vi "AttackerSmart.vi"(9 "balls":T1[](array[typedef])=[{"x"=-2165.869384765625, "y"=510.4085693359375, "timestamp"=timestamp(2082758857.4639893 s since 1904-01-01)}], 10 "Field Size in":T4={"line_width"=10, "field_length"=6000, "field_width"=4000, "boundary_width"=250, "referee_width"=425, "goal_width"=700, "goal_depth"=180, "goal_wall_width"=20, "center_circle_radius"=500, "defense_radius"=500, "defense_stretch"=350, "free_kick_from_defense_dist"=700, "penalty_spot_from_field_line_dist"=450, "penalty_line_from_spot_dist"=350}, 11 "Robot in":T2={"id"=5, "function"=enum."Attacker", "x"=-1842.5054931640625, "y"=520.60986328125, "orientation"=-2.7555055618286133, "v_tangent"=0.0, "v_normal"=0.0, "v_ang"=0.0, "kick_x"=0.0, "kick_z"=0.0, "dribble"=FALSE, "Timestamp"=timestamp(2082758857.4639893 s since 1904-01-01), "dest_x"=0.0, "dest_y"=0.0, "dest_orientation"=0.0}) -> (3 "Robot out":T2={"id"=5, "function"=enum."Attacker", "x"=-1842.5054931640625, "y"=520.60986328125, "orientation"=-2.7555055618286133, "v_tangent"=-0.08361641967936218, "v_normal"=-0.20513016702014014, "v_ang"=0.24456003022714357, "kick_x"=0.0, "kick_z"=0.0, "dribble"=FALSE, "Timestamp"=timestamp(2082758857.4639893 s since 1904-01-01), "dest_x"=0.0, "dest_y"=0.0, "dest_orientation"=0.0})   [LabVIEW 2016]
uses:
  Core/Field Size.ctl
  Core/AI Robot.ctl
  Functions Enum.ctl
  Core/AI Ball.ctl
  <vilib>/Analysis/coordinate.llb/Wrap Angle (scalar).vi
  <vilib>/Analysis/coordinate.llb/2D Cartesian Coordinate Rotation (Scalar).vi
  <vilib>/Analysis/NI_AALPro.lvlib
  <vilib>/Analysis/NI_AAL_Angle.lvlib
panel:
  in  "min ang to kick":dbl=0.09 format="%#_13g"
  in  "min dist to kick":dbl=195.0 format="%#_13g"
  in  "farback":dbl=330.0 format="%#_13g"
  in  "behind ball\ntarget aperture":dbl=0.3490658503988659 format="%#_13g"
  in  "conditional\nangle":dbl=0.45 format="%#_13g"
  in  "Kick Time":u32
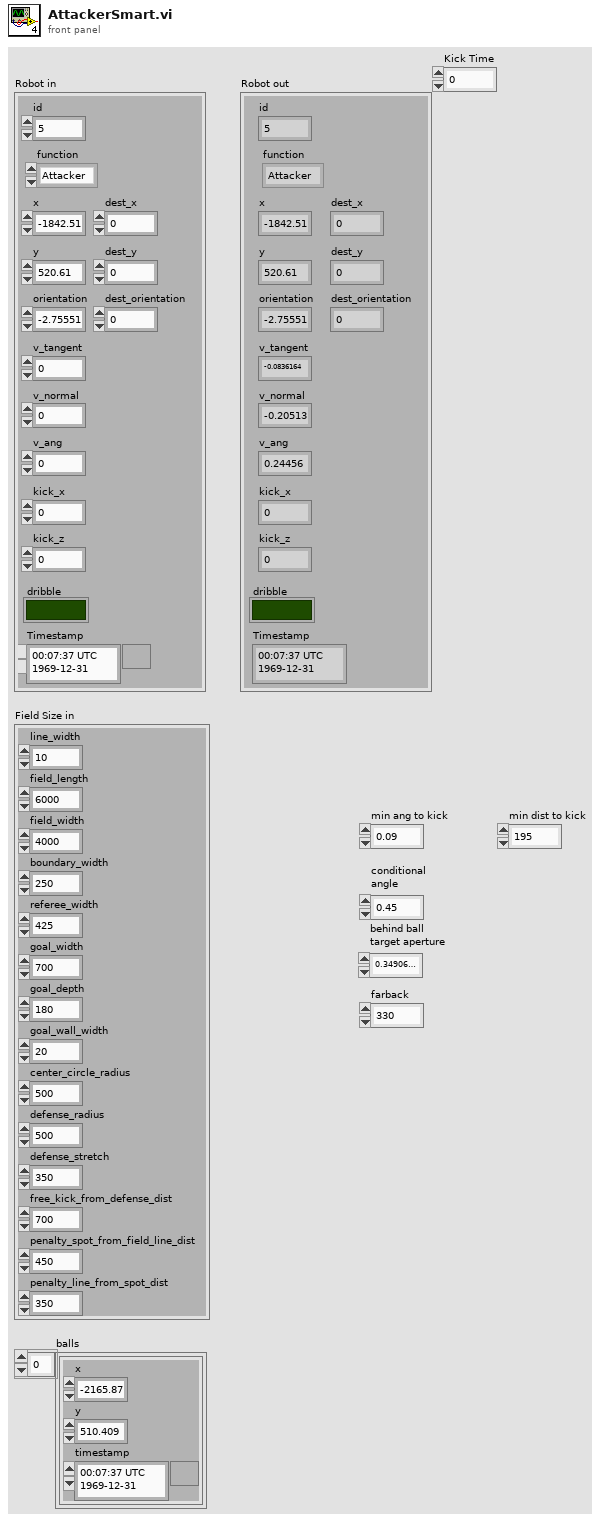
[diagram p1: front panel]
types:
  T1 = typedef "AI Ball.ctl" = cluster{"x":dbl, "y":dbl, "timestamp":timestamp}
  T2 = typedef "AI Robot.ctl" = cluster{"id":u32, "function":T3, "x":dbl, "y":dbl, "orientation":dbl, "v_tangent":dbl, "v_normal":dbl, "v_ang":dbl, "kick_x":dbl, "kick_z":dbl, "dribble":bool, "Timestamp":timestamp, "dest_x":dbl, "dest_y":dbl, "dest_orientation":dbl}
  T3 = typedef "Functions Enum.ctl" = enum16{"Attacker", "Goalie", "Defender", "Goto 0", "Dummy", "TDP"}
  T4 = typedef "Field Size.ctl" = cluster{"line_width":u32, "field_length":u32, "field_width":u32, "boundary_width":u32, "referee_width":u32, "goal_width":u32, "goal_depth":u32, "goal_wall_width":u32, "center_circle_radius":u32, "defense_radius":u32, "defense_stretch":u32, "free_kick_from_defense_dist":u32, "penalty_spot_from_field_line_dist":u32, "penalty_line_from_spot_dist":u32}
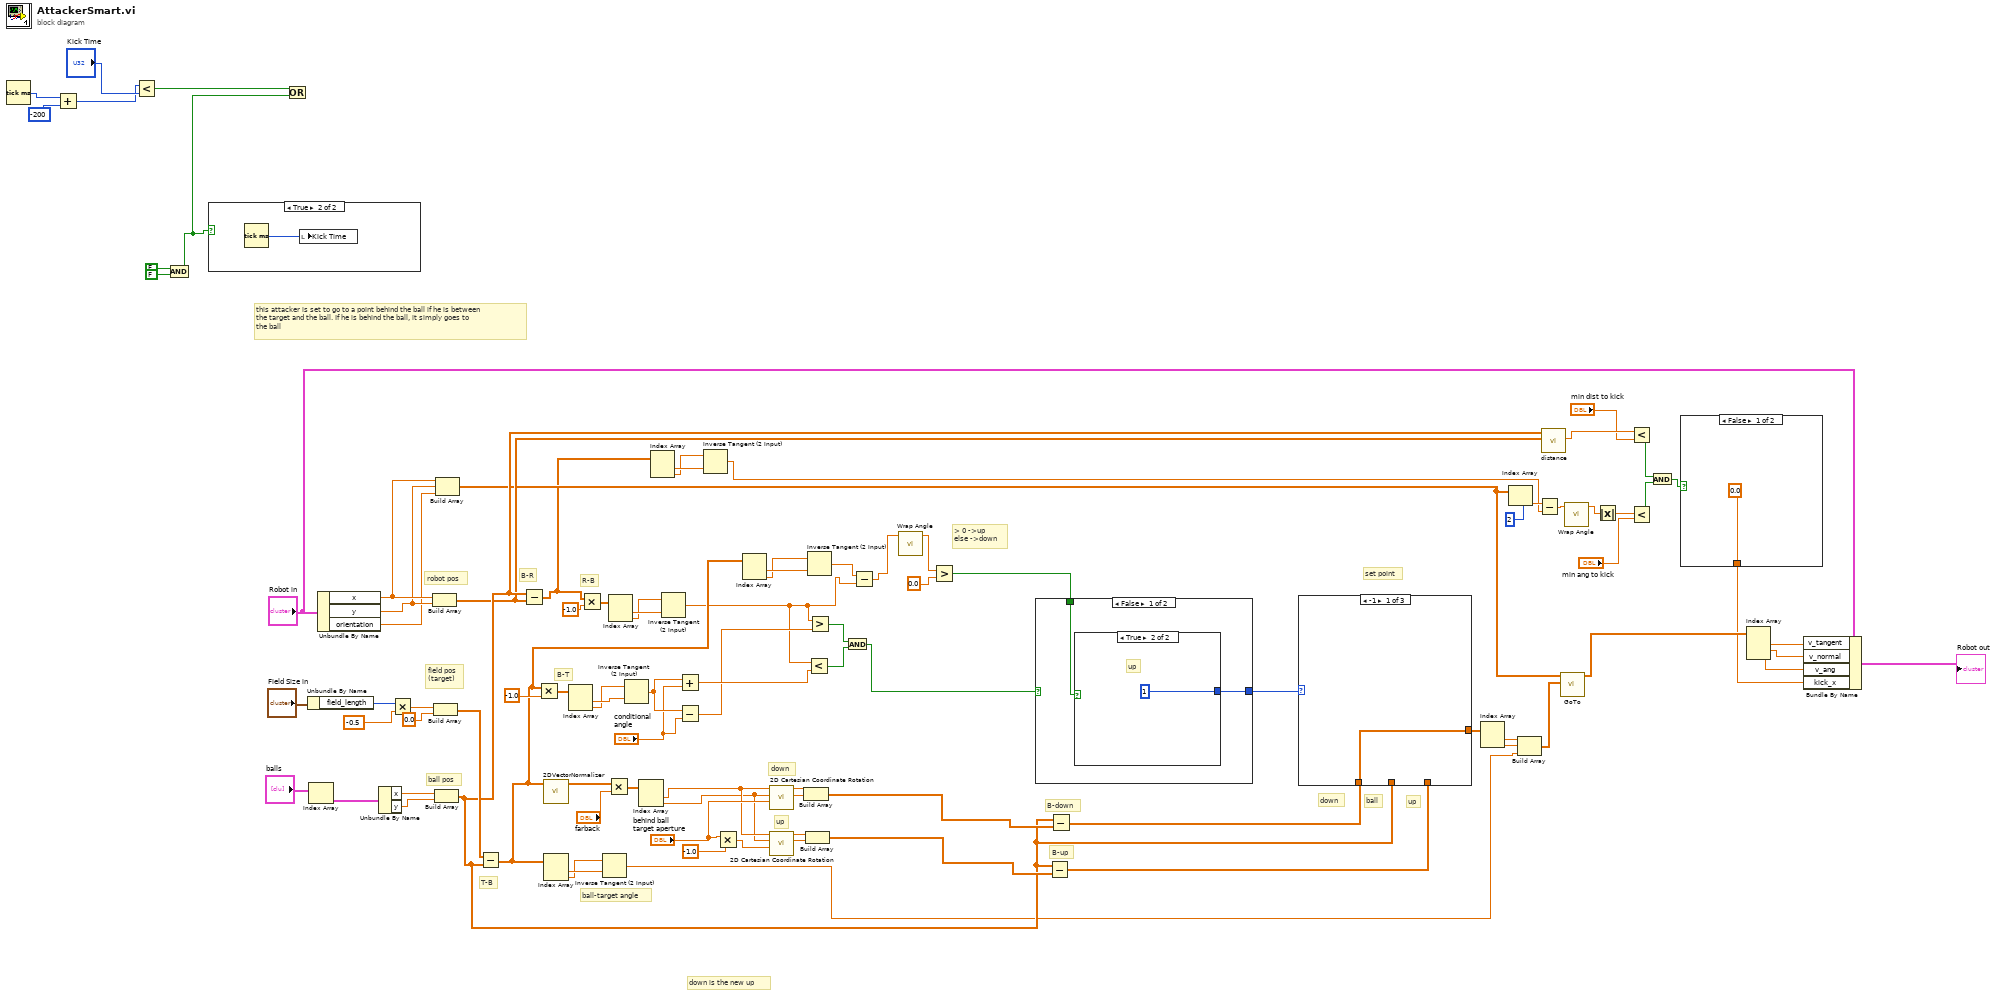
[diagram p0: block diagram]
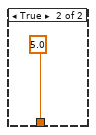
[diagram p2: hidden frame]
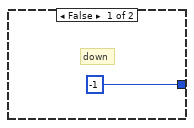
[diagram p5: hidden frame]
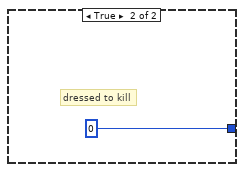
[diagram p6: hidden frame]
diagram:
  # "up"
  # "ball"
  # "down"
  # "set point"
  # "B-up"
  # "B-down"
  # "> 0 ->up\nelse ->down"
  # "down is the new up"
  # "B-T"
  # "T-B"
  # "R-B"
  # "B-R"
  # "up"
  # "down"
  # "ball-target angle"
  # "this attacker is set to go to a point behind the ball if he is between\nthe target and the ball. If he is behind the ball, it simply goes to\nthe ball"
  # "robot pos"
  # "field pos\n(target)"
  # "ball pos"
  n1 = Tick Count (ms)() -> (millisecond timer value=w94:u32)
  n2 = Add(x=w94, y=-200) -> (x+y=w91:u32)
  n3 = Less?(x=w91, y="Kick Time") -> (x < y?=w90:bool)
  n4 = And(x=FALSE, y=FALSE) -> (x .and. y?=w89:bool)
  n5 = case shown="True" w89 {
    frame False {
    }
    frame True {
      n6 = Tick Count (ms)() -> (millisecond timer value=w95:u32)
      n7 = local write "Kick Time"(w95) -> ()
    }
  }
  n8 = Or(x=w90, y=w89) -> ()  [unwired: 1 out]
  n9 = Unbundle By Name("Field Size in") -> ("field_length"=w85:u32)
  n10 = Index Array(array="balls") -> (element=w87:T1)  [unwired: 1 in]
  n11 = Unbundle By Name("Robot in") -> ("x"=w33:dbl, "y"=w32:dbl, "orientation"=w31:dbl)
  n12 = Unbundle By Name(w87) -> ("x"=w81:dbl, "y"=w80:dbl)
  n13 = Multiply(x=w85, y=-0.5) -> (x*y=w83:dbl)
  n14 = Build Array(w33, w32) -> (w25:dbl[])
  n15 = Build Array(w83, 0.0 ("element")) -> (w79:dbl[])
  n16 = Build Array(w81, w80) -> (w26:dbl[])
  n17 = Build Array(w33, w32, w31) -> (w22:dbl[])
  n18 = Subtract(x=w79, y=w26) -> (x-y=w45:dbl[])
  n19 = Subtract(x=w26, y=w25) -> (x-y=w2:dbl[])
  n20 = Multiply(x=w45, y=-1.0) -> (x*y=w55:dbl[])
  n21 = call "2DVectorNormalizer.vi"("2D vector"=w45) -> ("2D vector 2"=w74:dbl[])  [unwired: 10 in]
  n22 = Index Array(array=w45) -> (element #1=w78:dbl, element #2=w77:dbl)  [unwired: 2 in]
  n23 = Index Array(array=w55) -> (element #1=w57:dbl, element #2=w56:dbl)  [unwired: 2 in]
  n24 = Multiply(x=w2, y=-1.0) -> (x*y=w59:dbl[])
  n25 = Inverse Tangent (2 Input)(1:w78, 2:w77) -> (0:w19:dbl)
  n26 = Multiply(x=w74, y="farback") -> (x*y=w72:dbl[])
  n27 = Index Array(array=w59) -> (element #1=w61:dbl, element #2=w60:dbl)  [unwired: 2 in]
  n28 = Inverse Tangent (2 Input)(1:w57, 2:w56) -> (0:w54:dbl)
  n29 = Index Array(array=w72) -> (element #1=w66:dbl, element #2=w65:dbl)  [unwired: 2 in]
  n30 = Index Array(array=w2) -> (element #1=w4:dbl, element #2=w3:dbl)  [unwired: 2 in]
  n31 = Inverse Tangent (2 Input)(1:w61, 2:w60) -> (0:w39:dbl)
  n32 = Add(x=w54, y="conditional\nangle") -> (x+y=w52:dbl)
  n33 = Subtract(x=w54, y="conditional\nangle") -> (x-y=w51:dbl)
  n34 = Inverse Tangent (2 Input)(1:w4, 2:w3) -> (0:w1:dbl)
  n35 = Multiply(x="behind ball\ntarget aperture", y=-1.0) -> (x*y=w67:dbl)
  n36 = Index Array(array=w45) -> (element #1=w47:dbl, element #2=w46:dbl)  [unwired: 2 in]
  n37 = call-poly <vilib>:"2D Cartesian Coordinate Rotation.vi"("theta"="behind ball\ntarget aperture", "y"=w65, "x"=w66) -> ("y out"=w70:dbl, "x out"=w71:dbl)  [unwired: 6 in, 1 out]
  n38 = call-poly <vilib>:"2D Cartesian Coordinate Rotation.vi"("theta"=w67, "y"=w65, "x"=w66) -> ("y out"=w63:dbl, "x out"=w64:dbl)  [unwired: 6 in, 1 out]
  n39 = Build Array(w71, w70) -> (w38:dbl[])
  n40 = Build Array(w64, w63) -> (w37:dbl[])
  n41 = Inverse Tangent (2 Input)(1:w47, 2:w46) -> (0:w40:dbl)
  n42 = Less?(x=w39, y=w52) -> (x < y?=w49:bool)
  n43 = Greater?(x=w39, y=w51) -> (0:w50:bool)
  n44 = And(x=w50, y=w49) -> (x .and. y?=w48:bool)
  n45 = Subtract(x=w40, y=w39) -> (x-y=w42:dbl)
  n46 = call-poly <vilib>:"Wrap Angle.vi"("angle in"=w42) -> ("angle out"=w41:dbl)  [unwired: 9 in, 1 out]
  n47 = Greater?(x=w41, y=0.0) -> (0:w43:bool)
  n48 = case shown="False" w48 {
    tunnel: [w96 0] -> w36
    tunnel: w43 -> [w97 _]
    frame False {
      n49 = case shown="True" w97 {
        tunnel: [-1 1] -> w96
        frame False {
          # "down"
        }
        frame True {
          # "up"
        }
      }
    }
    frame True {
      # "dressed to kill"
    }
  }
  n50 = Subtract(x=w26, y=w37) -> (x-y=w34:dbl[])
  n51 = Subtract(x=w26, y=w38) -> (x-y=w35:dbl[])
  n52 = case shown="-1" w36 {
    tunnel: w35 -> [w101 _ _]
    tunnel: w34 -> [_ _ w103]
    tunnel: w26 -> [_ w102 _]
    tunnel: [w101 w102 w103] -> w30
    frame -1 {
    }
    frame 0, Default {
    }
    frame 1 {
    }
  }
  n53 = Index Array(array=w30) -> (element #1=w29:dbl, element #2=w28:dbl)  [unwired: 2 in]
  n54 = Index Array(array=w22, index=2) -> (element=w20:dbl)
  n55 = Build Array(w29, w28, w19) -> (w27:dbl[])
  n56 = Subtract(x=w20, y=w1) -> (x-y=w18:dbl)
  n57 = call "distance.vi"("target pos"=w25, "obj pos"=w26) -> ("sqrt(x)"=w24:dbl)  [unwired: 9 in]
  n58 = call "GoTo.vi"("Target"=w27, "Position"=w22) -> ("Output\nVelocity"=w12:dbl[])  [unwired: 9 in]
  n59 = call-poly <vilib>:"Wrap Angle.vi"("angle in"=w18) -> ("angle out"=w17:dbl)  [unwired: 9 in, 1 out]
  n60 = Absolute Value(x=w17) -> (abs(x)=w16:dbl)
  n61 = Less?(x=w24, y="min dist to kick") -> (x < y?=w7:bool)
  n62 = Less?(x=w16, y="min ang to kick") -> (x < y?=w6:bool)
  n63 = And(x=w7, y=w6) -> (x .and. y?=w8:bool)
  n64 = case shown="False" w8 {
    tunnel: [0.0 5.0] -> w5
    frame False {
    }
    frame True {
    }
  }
  n65 = Index Array(array=w12) -> (element #1=w11:dbl, element #2=w10:dbl, element #3=w9:dbl)  [unwired: 3 in]
  n66 = Bundle By Name(cluster="Robot in", "v_tangent"=w11, "v_normal"=w10, "v_ang"=w9, "kick_x"=w5) -> (→"Robot out":T2)
